vi "ABOUT SCREEN config read.vi"(8 "error in (no error)":errorcluster) -> (0 "error out":errorcluster, 3 "ABOUT SCREEN Parameters":string[](array[string]))   [LabVIEW 2025]
uses:
  Configuraton Files/Config file  FGV Unitest enum.ctl
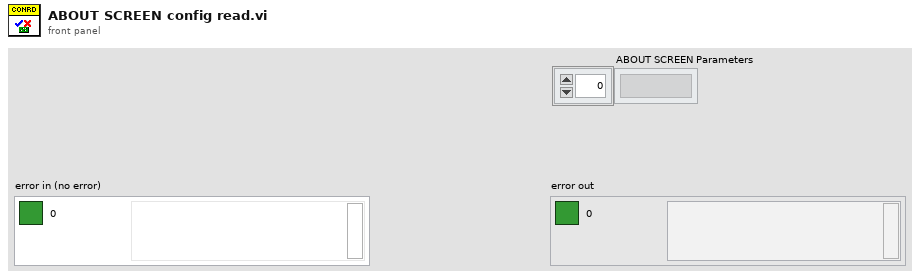
[diagram p1: front panel]
types:
  T1 = typedef "Config file  FGV Unitest enum.ctl" = enum16{"OPEN", "READ", "WRITE", "CLOSE"}
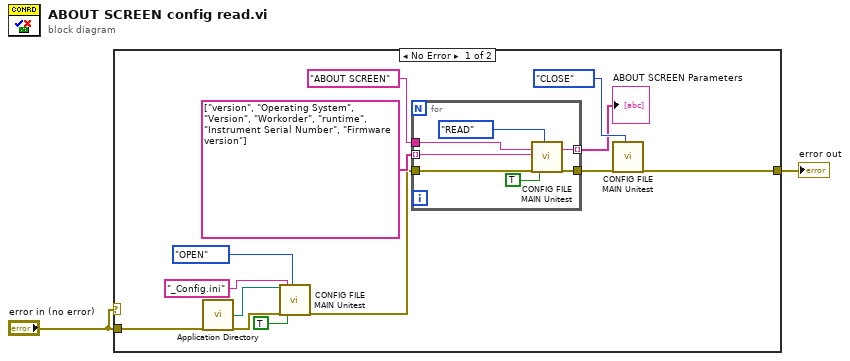
[diagram p0: block diagram]
diagram:
  n1 = case shown="No Error" "error in (no error)" {
    tunnel: [w14 _] -> w2
    tunnel: "error in (no error)" -> [w9 _]
    frame No Error {
      n2 = call <vilib>:"Application Directory.vi"() -> ("Application Directory"=w6:path)
      n3 = call "CONFIG FILE MAIN Unitest.vi"("File Path"=w6, "error in"=w9, "file name"="_Config.ini", "PARAMETER/CONFIG"=TRUE, "Config Enum"=Config_file__FGV_Unitest_enum."OPEN") -> ("error out"=w4:errorcluster)  [unwired: 13 in, 1 out]
      n4 = for {
        tunnel: "ABOUT SCREEN" ("WRITE /READ SECTION") -> [w21]
        tunnel: [w20] -> w11
        tunnel: string[] ["version", "Operating System", "Version", "Workorder", "runtime", "Instrument Serial Number", "Firmware version"] -> [w17] mode=indexing
        tunnel: [w16] -> w3 mode=indexing
        tunnel: w4 -> [w15]
        n5 = call "CONFIG FILE MAIN Unitest.vi"("WRITE /READ SECTION"=w21, "READ KEY"=w17, "error in"=w15, "PARAMETER/CONFIG"=TRUE, "Config Enum"=Config_file__FGV_Unitest_enum."READ") -> ("READ VALUE"=w16:string, "error out"=w20:errorcluster)  [unwired: 13 in]
      }
      "ABOUT SCREEN Parameters" <- w3
      n6 = call "CONFIG FILE MAIN Unitest.vi"("error in"=w11, "Config Enum"=Config_file__FGV_Unitest_enum."CLOSE") -> ("error out"=w14:errorcluster)  [unwired: 16 in, 1 out]
    }
    frame Error {
    }
  }
  "error out" <- w2
